vi "X Errors Read.vi"(4 "error in (no error)":errorcluster, 6 "Container State":T2, 7 "Display State In":T1) -> (0 "error out":errorcluster, 2 "Value":dbl[](array[numeric]), 3 "Display State Out":T1)   [LabVIEW 2018, in "XY Plot with Error Bars.xctl"]
uses:
  XY Plot with Error Bars.xctl
  <vilib>/_xctls/Container State.ctl
  State.ctl
  <vilib>/_xctls/XControlSupport.lvlib
panel:
  # "Replace the Value Indicator below with an Indicator of desired type.\nDo not remove this Indicator or the others from the connector pane. \nDo not change the connector pane pattern.\nThe Value Indicator should always be the second terminal from top on the output side in the connector pane."
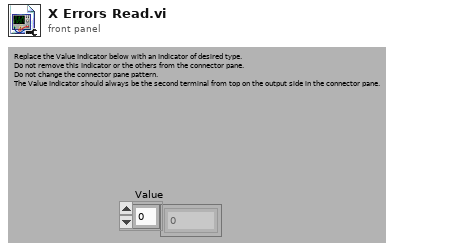
[diagram p1: front panel]
types:
  T1 = typedef "XY Plot with Error Bars.xctl/State.ctl" = cluster{"XCTLRefs":refnum<vi>[], "Delta X":dbl[], "Delta Y":dbl[]}
  T2 = typedef "XControlSupport.lvlib/Container State.ctl" = cluster{"Indicator?":bool, "Run Mode?":bool, " Refnum":refnum<vi>}
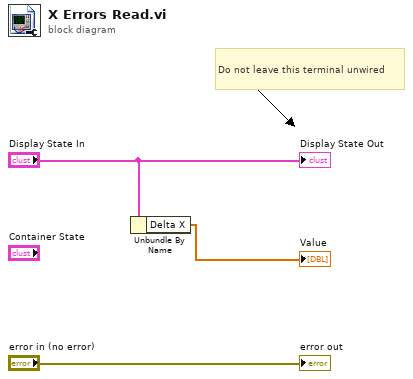
[diagram p0: block diagram]
diagram:
  # "Do not leave this terminal unwired"
  n1 = Unbundle By Name("Display State In") -> ("Delta X"=→"Value":dbl[])
  "error out" <- "error in (no error)"
  "Display State Out" <- "Display State In"
